vi "Channel Type.vi"() -> (2 "Channel Template":string)   [LabVIEW 2022 SP3, in "FlexBlocks Support.lvlib"]
uses:
  FlexBlocks Support.lvlib
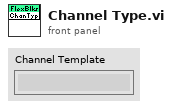
[diagram p1: front panel]
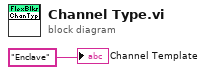
[diagram p0: block diagram]
diagram:
  "Channel Template" <- "Enclave" ("Channel Template")
